vi "is over connection limit.vi"(7 "precheck?":bool, 11 "connection server in":refnum<class "connection server.lvclass">) -> (3 "over limit?":bool)   [LabVIEW 2015, in "connection server.lvclass"]
uses:
  connection server.lvclass
  connection server.lvclass/connection server.ctl
  communicator/communicator.lvclass
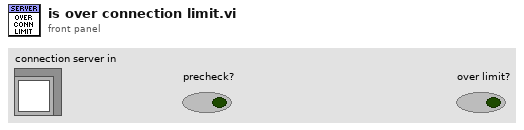
[diagram p1: front panel]
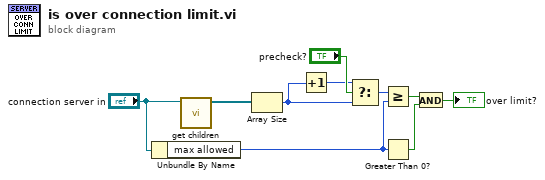
[diagram p0: block diagram]
diagram:
  n1 = Unbundle By Name("connection server in") -> ("max allowed"=w8:i32)
  n2 = call "get children.vi"("communicator in"="connection server in") -> ("children"=w5:refnum<class "identifying queue.lvclass">[])  [unwired: 10 in]
  n3 = Array Size(array=w5) -> (size(s)=w1:i32)
  n4 = Increment(x=w1) -> (x+1=w2:i32)
  n5 = Select(t=w2, s="precheck?", f=w1) -> (s? t:f=w3:i32)
  n6 = Greater Or Equal?(x=w3, y=w8) -> (x >= y?=w9:bool)
  n7 = Greater Than 0?(x=w8) -> (x > 0?=w10:bool)
  n8 = And(x=w9, y=w10) -> (x .and. y?=→"over limit?":bool)
